vi "LastStepMsgParser.vi"(6 "Arr Refnum":refnum<vi>, 7 "Out MSG Names":string[](array[string]), 8 "old msg counter":i32, 9 "Codes":i32[](array[numeric]), 10 "Msg Array":T1(array[cluster])) -> (2 "code":i32[](array[numeric]), 3 "current msg counter":i32)   [LabVIEW 2010]
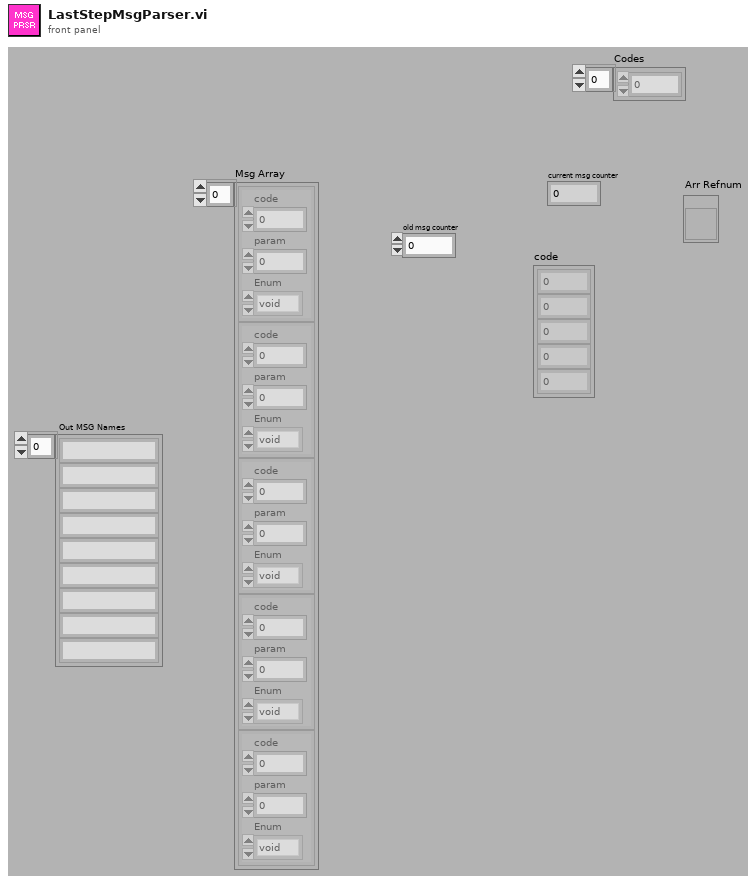
[diagram p1: front panel]
types:
  T1 = cluster{"code":i32, "param":i32, "Enum":enum16{"void", "byte", "int", "float"}}[]
  T2 = cluster{"code":i32, "param":i32, "Enum":enum16{"void", "byte", "int", "float"}}
  T3 = cluster{"Сообщение":string, "Значение":string, "Тип":enum16{"void", "byte", "int", "float"}}[]
  T4 = cluster{"Сообщение":string, "Значение":string, "Тип":enum16{"void", "byte", "int", "float"}}
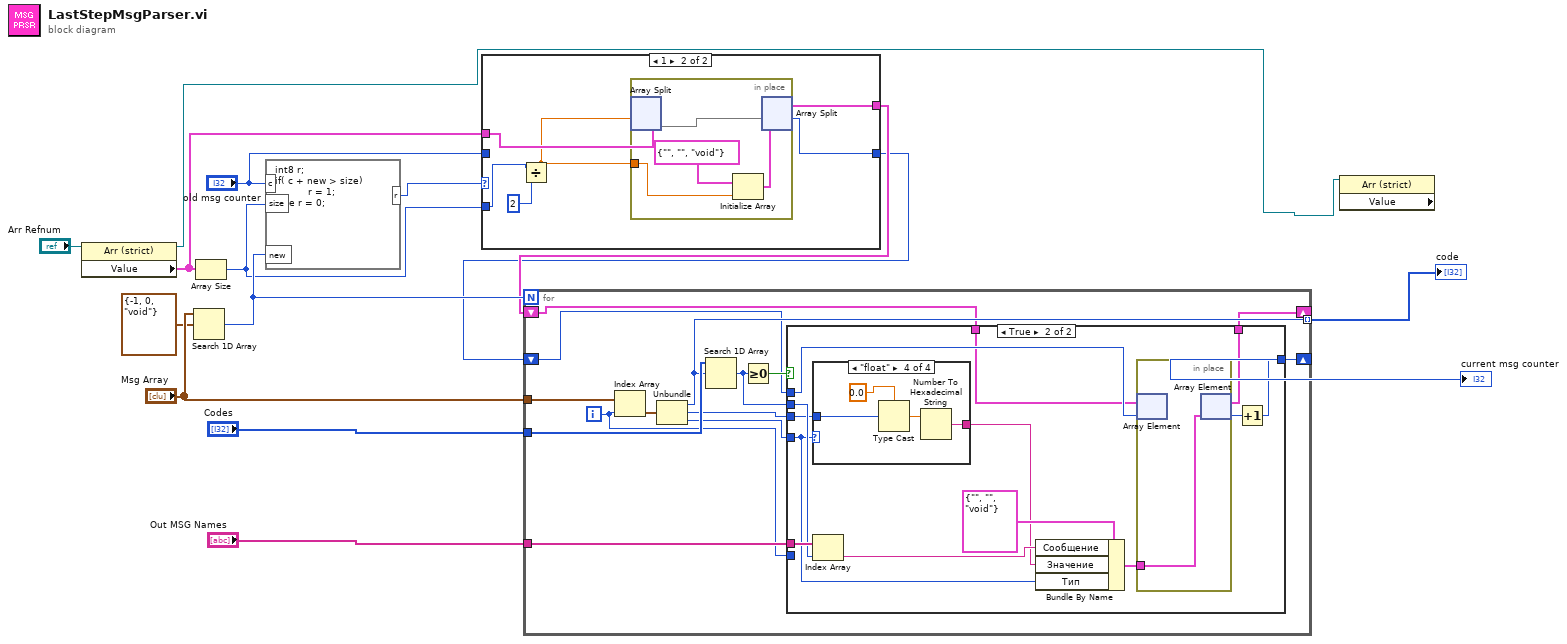
[diagram p0: block diagram]
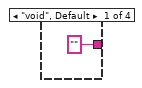
[diagram p4: hidden frame]
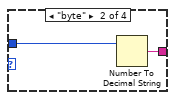
[diagram p5: hidden frame]
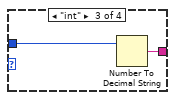
[diagram p6: hidden frame]
diagram:
  n1 = property class="Arr (strict)"(reference="Arr Refnum") -> (reference out=w4:refnum<vi>, "Value"=w7:T3)  [unwired: 1 in, 1 out]
  n2 = Search 1D Array(1D array="Msg Array", element=T2 {"code"=-1, "param"=0, "Enum"=enum."void"} ("Cluster")) -> (index of element=w6:i32)  [unwired: 1 in]
  n3 = Array Size(array=w7) -> (size(s)=w3:i32)
  n4 = formula code="int8 r;\nif( c + new > size)\n           r = 1;\nelse r = 0;"("c"="old msg counter", "size"=w3, "new"=w6) -> ("r"=w8:i8)
  n5 = case shown="1" w8 {
    tunnel: w7 -> [w17 w21]
    tunnel: w3 -> [_ w23]
    tunnel: [w17 w19] -> w5
    tunnel: "old msg counter" -> [w16 _]
    tunnel: [w16 w18] -> w1
    frame 0, Default {
    }
    frame 1 {
      n6 = Divide(x=w23, y=2) -> (x/y=w20:dbl)
      n7 = in-place {
        in-place-border: w20 -> [w26]
        n8 = in-place-split #1(w21, w20) -> (w27:T3)  [unwired: 1 out]
        n9 = Initialize Array(T4 {"Сообщение"="", "Значение"="", "Тип"=enum."void"} ("Cluster"), w26) -> (w24:T3)
        n10 = in-place-split #1(w27, w24) -> (w19:T3, w18:i32)
      }
    }
  }
  n11 = for {
    N: w6 -> [_]
    tunnel: "Msg Array" -> [w36]
    tunnel: [w32] -> w14 mode=indexing
    tunnel: "Codes" -> [w39]
    tunnel: "Out MSG Names" -> [w38]
    shift-right: [w30] -> w10
    shift-left: w1 -> [w31]
    shift-right: [w28] -> _
    shift-left: w5 -> [w29]
    i -> [w35]
    n12 = Index Array(array=w36, index=w35) -> (element=w34:T2)
    n13 = Unbundle(w34) -> ("code"=w32:i32, "param"=w37:i32, "Enum"=w33:enum16{"void", "byte", "int", "float"})
    n14 = Search 1D Array(1D array=w39, element=w32) -> (index of element=w40:i32)  [unwired: 1 in]
    n15 = Greater Or Equal To 0?(x=w40) -> (x >= 0?=w41:bool)
    n16 = case shown="True" w41 {
      tunnel: w38 -> [_ w56]
      tunnel: w40 -> [_ w55]
      tunnel: w37 -> [_ w54]
      tunnel: w35 -> [_ _]
      tunnel: w33 -> [_ w50]
      tunnel: w31 -> [w43 w47]
      tunnel: [w43 w48] -> w30
      tunnel: w29 -> [w42 w46]
      tunnel: [w42 w45] -> w28
      frame False {
      }
      frame True {
        n17 = case shown="\"float\"" w50 {
          tunnel: w54 -> [_ w60 w62 w66]
          tunnel: ["" ("decimal integer string") w59 w61 w63] -> w51
          frame "void", Default {
          }
          frame "byte" {
            n18 = Number To Decimal String(number=w60) -> (decimal integer string=w59:string)  [unwired: 1 in]
          }
          frame "int" {
            n19 = Number To Decimal String(number=w62) -> (decimal integer string=w61:string)  [unwired: 1 in]
          }
          frame "float" {
            n20 = Type Cast(type=0.0 ("default (0 dbl)"), x=w66) -> (*(type *) &x=w64:dbl)
            n21 = Number To Hexadecimal String(2:w64) -> (0:w63:string)  [unwired: 1 in]
          }
        }
        n22 = Index Array(array=w56, index=w55) -> (element=w52:string)
        n23 = Bundle By Name(cluster=T4 {"Сообщение"="", "Значение"="", "Тип"=enum."void"} ("Cluster"), "Сообщение"=w52, "Значение"=w51, "Тип"=w50) -> (w49:T4)
        n24 = in-place {
          in-place-border: w49 -> [w57]
          n25 = in-place-array #2(w46, w47) -> ()  [unwired: 1 out]
          n26 = in-place-array #2(w57) -> (w45:T3, w44:i32)
        }
        n27 = Increment(x=w44) -> (x+1=w48:i32)
      }
    }
  }
  "code" <- w14
  "current msg counter" <- w10
  n28 = property class="Arr (strict)" props=["Value"](reference=w4) -> ()  [unwired: 1 in, 3 out]
